vi "质控启动参数选择对话框.vi"(8 "COD":bool, 9 "总氮":bool, 10 "总磷":bool, 11 "氨氮":bool) -> (1 "取消启动":bool, 2 "确定启动":bool, 3 "启动模块":T1)   [LabVIEW 2016, in "质控单元.lvlib"]
panel:
  in  "总氮":bool
  in  "确定":bool
  in  "COD":bool
  in  "总磷":bool
  in  "取消":bool
  in  "氨氮":bool
  # "请选择加标回收模块"
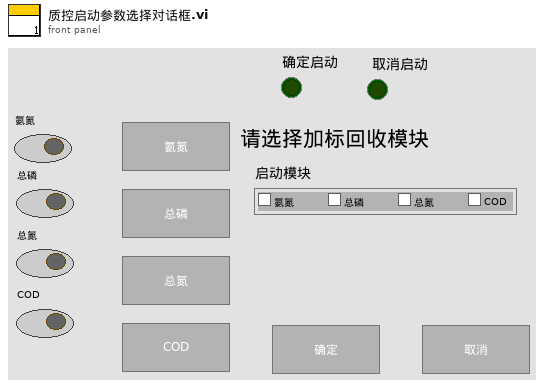
[diagram p1: front panel]
types:
  T1 = cluster{"氨氮":bool, "总磷":bool, "总氮":bool, "COD":bool}
  T2 = cluster{"氨氮1":bool, "总磷1":bool, " COD1":bool, "总磷1 2":bool}
  T3 = cluster{"氨氮1":bool, "总磷1":bool, "总氮":bool, " COD1":bool}
  T4 = enum8{"Enabled", "Disabled", "Disabled and Grayed Out"}
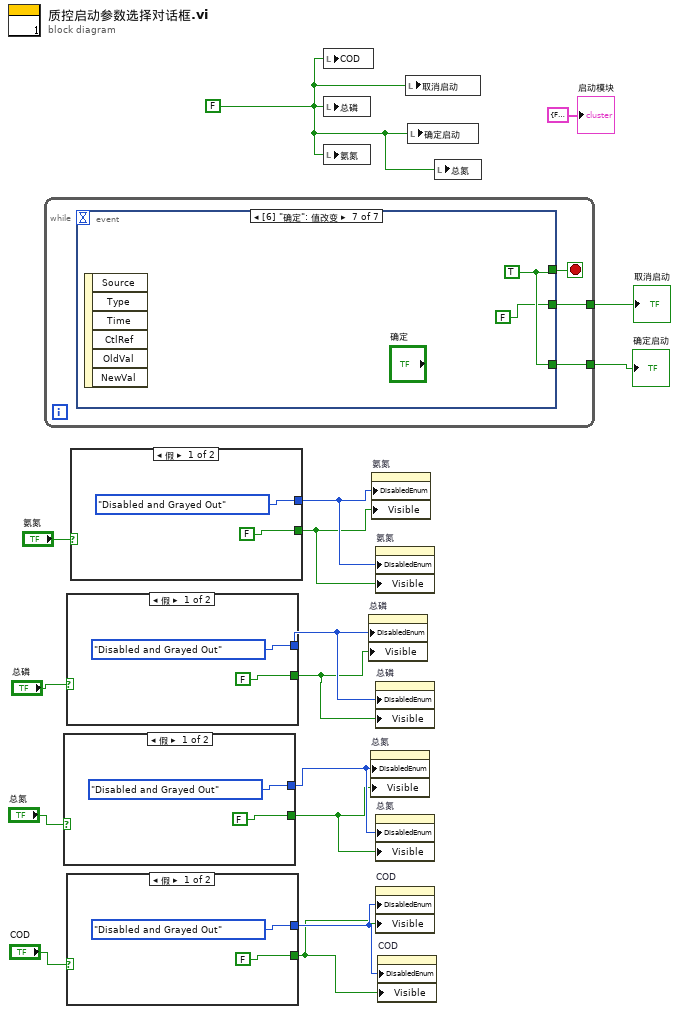
[diagram p0: block diagram]
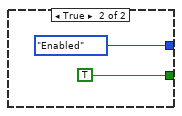
[diagram p2: hidden frame]
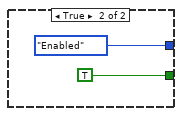
[diagram p3: hidden frame]
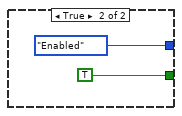
[diagram p4: hidden frame]
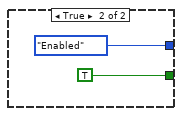
[diagram p5: hidden frame]
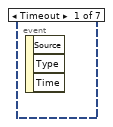
[diagram p6: hidden frame]
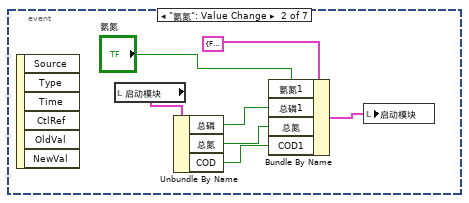
[diagram p7: hidden frame]
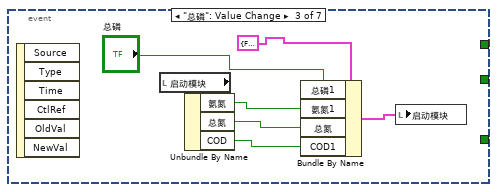
[diagram p8: hidden frame]
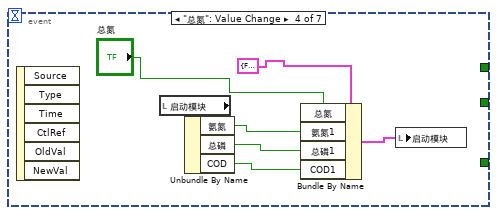
[diagram p9: hidden frame]
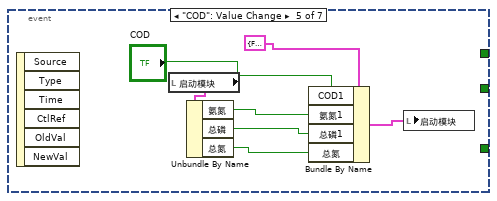
[diagram p10: hidden frame]
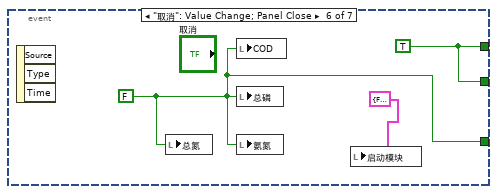
[diagram p11: hidden frame]
diagram:
  w13 = FALSE ("确定")
  n1 = while {
    tunnel: [w18] -> w16
    tunnel: [w17] -> w15
    stop <- w19 stop-if-true
    n2 = event shown="[6] \"确定\": 值改变" {
      selector: _ -> [_ _ _ _ _ _ _]
      dyn-events: _ -> [_ _ _ _ _ _ _]
      timeout: _ -> [_ _ _ _ _ _ _]
      tunnel: [_ _ _ _ _ w50 w52] -> w19
      tunnel: [_ _ _ _ _ w48 w52] -> w18
      tunnel: [_ _ _ _ _ w50 FALSE ("确定")] -> w17
      event Timeout {
        n3 = event-data() -> ()  [unwired: 1 in, 3 out]
      }
      event "氨氮": Value Change {
        n4 = event-data() -> ()  [unwired: 1 in, 6 out]
        n5 = local read "启动模块"() -> (w25:T1)
        n6 = Unbundle By Name(w25) -> ("总磷"=w24:bool, "总氮"=w23:bool, "COD"=w21:bool)
        n7 = Bundle By Name(cluster=T3 {"氨氮1"=FALSE, "总磷1"=FALSE, "总氮"=FALSE, " COD1"=FALSE} ("启动模块"), "氨氮1"="氨氮", "总磷1"=w24, "总氮"=w23, "COD1"=w21) -> (w20:T3)
        n8 = local write "启动模块"(w20) -> ()
      }
      event "总磷": Value Change {
        n9 = event-data() -> ()  [unwired: 1 in, 6 out]
        n10 = local read "启动模块"() -> (w33:T1)
        n11 = Unbundle By Name(w33) -> ("氨氮"=w32:bool, "总氮"=w31:bool, "COD"=w27:bool)
        n12 = Bundle By Name(cluster=T3 {"氨氮1"=FALSE, "总磷1"=FALSE, "总氮"=FALSE, " COD1"=FALSE} ("启动模块"), "总磷1"="总磷", "氨氮1"=w32, "总氮"=w31, "COD1"=w27) -> (w30:T3)
        n13 = local write "启动模块"(w30) -> ()
      }
      event "总氮": Value Change {
        n14 = event-data() -> ()  [unwired: 1 in, 6 out]
        n15 = local read "启动模块"() -> (w40:T1)
        n16 = Unbundle By Name(w40) -> ("氨氮"=w39:bool, "总磷"=w38:bool, "COD"=w35:bool)
        n17 = Bundle By Name(cluster=T3 {"氨氮1"=FALSE, "总磷1"=FALSE, "总氮"=FALSE, " COD1"=FALSE} ("启动模块"), "总氮"="总氮", "氨氮1"=w39, "总磷1"=w38, "COD1"=w35) -> (w37:T3)
        n18 = local write "启动模块"(w37) -> ()
      }
      event "COD": Value Change {
        n19 = event-data() -> ()  [unwired: 1 in, 6 out]
        n20 = local read "启动模块"() -> (w47:T1)
        n21 = Unbundle By Name(w47) -> ("氨氮"=w46:bool, "总磷"=w45:bool, "总氮"=w41:bool)
        n22 = Bundle By Name(cluster=T3 {"氨氮1"=FALSE, "总磷1"=FALSE, "总氮"=FALSE, " COD1"=FALSE} ("启动模块"), "COD1"="COD", "氨氮1"=w46, "总磷1"=w45, "总氮"=w41) -> (w44:T3)
        n23 = local write "启动模块"(w44) -> ()
      }
      event "取消": Value Change; Panel Close {
        w48 = FALSE ("确定")
        w50 = TRUE ("确定")
        n24 = event-data() -> ()  [unwired: 1 in, 3 out]
        n25 = local write "总氮"(w48) -> ()
        n26 = local write "COD"(w48) -> ()
        n27 = local write "总磷"(w48) -> ()
        n28 = local write "氨氮"(w48) -> ()
        n29 = local write "启动模块"(T2 {"氨氮1"=FALSE, "总磷1"=FALSE, " COD1"=FALSE, "总磷1 2"=FALSE} ("启动模块")) -> ()
      }
      event "确定": Value Change {
        w52 = TRUE ("确定")
        n30 = event-data() -> ()  [unwired: 1 in, 6 out]
      }
    }
  }
  "确定启动" <- w16
  "取消启动" <- w15
  n31 = case shown="假" "总氮" {
    tunnel: [T4."Disabled and Grayed Out" ("禁用") T4."Enabled" ("禁用")] -> w4
    tunnel: [FALSE ("可见") TRUE ("可见")] -> w3
    frame False {
    }
    frame True {
    }
  }
  n32 = case shown="假" "总磷" {
    tunnel: [T4."Disabled and Grayed Out" ("禁用") T4."Enabled" ("禁用")] -> w6
    tunnel: [FALSE ("可见") TRUE ("可见")] -> w5
    frame False {
    }
    frame True {
    }
  }
  n33 = case shown="假" "COD" {
    tunnel: [T4."Disabled and Grayed Out" ("禁用") T4."Enabled" ("禁用")] -> w2
    tunnel: [FALSE ("可见") TRUE ("可见")] -> w1
    frame False {
    }
    frame True {
    }
  }
  n34 = case shown="假" "氨氮" {
    tunnel: [T4."Disabled and Grayed Out" ("禁用") T4."Enabled" ("禁用")] -> w8
    tunnel: [FALSE ("可见") TRUE ("可见")] -> w7
    frame False {
    }
    frame True {
    }
  }
  n35 = local write "COD"(w13) -> ()
  n36 = local write "总磷"(w13) -> ()
  n37 = local write "氨氮"(w13) -> ()
  n38 = property on="总磷" class="Bool (严格)"("DisabledEnum"=w6, "Visible"=w5) -> ()  [unwired: 2 in, 2 out]
  n39 = property on="总氮" class="Bool (严格)"("DisabledEnum"=w4, "Visible"=w3) -> ()  [unwired: 2 in, 2 out]
  n40 = property on="氨氮" class="Bool (严格)"("DisabledEnum"=w8, "Visible"=w7) -> ()  [unwired: 2 in, 2 out]
  n41 = property on="氨氮" class="Bool (严格)"("DisabledEnum"=w8, "Visible"=w7) -> ()  [unwired: 2 in, 2 out]
  n42 = property on="总磷" class="Bool (严格)"("DisabledEnum"=w6, "Visible"=w5) -> ()  [unwired: 2 in, 2 out]
  n43 = property on="总氮" class="Bool (严格)"("DisabledEnum"=w4, "Visible"=w3) -> ()  [unwired: 2 in, 2 out]
  n44 = property on="COD" class="Bool (严格)"("DisabledEnum"=w2, "Visible"=w1) -> ()  [unwired: 2 in, 2 out]
  n45 = property on="COD" class="Bool (严格)"("DisabledEnum"=w2, "Visible"=w1) -> ()  [unwired: 2 in, 2 out]
  n46 = local write "取消启动"(w13) -> ()
  n47 = local write "确定启动"(w13) -> ()
  n48 = local write "总氮"(w13) -> ()
  "启动模块" <- T2 {"氨氮1"=FALSE, "总磷1"=FALSE, " COD1"=FALSE, "总磷1 2"=FALSE} ("启动模块")
